vi "TDC_writeTimestamps.vi"(8 "Error In":errorcluster, 10 "binary Format":bool, 11 "Path":path) -> (0 "Error Out":errorcluster)   [LabVIEW 2011]
uses:
  dist/userlib/lib/tdcbase.dll
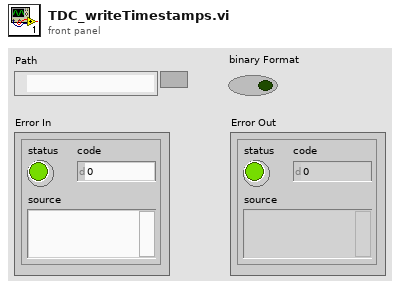
[diagram p1: front panel]
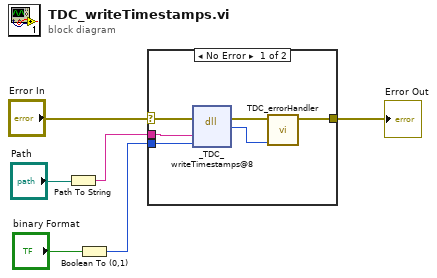
[diagram p0: block diagram]
diagram:
  n1 = Path To String(path="Path") -> (string=w1:string)
  n2 = Boolean To (0,1)(Boolean="binary Format") -> (0, 1=w3:i16)
  n3 = case shown="No Error" "Error In" {
    selector: "Error In" -> [w12 w13]
    tunnel: [w9 w13] -> w5
    tunnel: w3 -> [w8 _]
    tunnel: w1 -> [w7 _]
    frame No Error {
      n4 = dll-call lib="C:/nh/projekt/spmctrl/dist/userlib/lib/tdcbase.dll" fn="_TDC_writeTimestamps@8"(error in=w12, "filename"=w7, "binary"=w8) -> (error out=w11:errorcluster, "return type"=w10:i32)  [unwired: 4 in, 1 out]
      n5 = call "TDC_errorHandler.vi"("quTAU Return Code"=w10, "Error In"=w11) -> ("Error Out"=w9:errorcluster)  [unwired: 9 in]
    }
    frame Error {
    }
  }
  "Error Out" <- w5
